vi "generate wave packet V3.vi"(7 "number of grid points":i32=300, 9 "z window":dbl=3.0, 11 "wavepacket in":T1={"R"=0.5, "wave number"=22.0, "delta k"=7.0, "radii vector"=[], "radial section"=[], "wave vector"=22.0, "wavepacket is"=TRUE} {"delta k" format="%#_3f"; "wave number" format="%#_3f"; "R" format="%#_3f"}) -> (1 "pond array out":cdb[][](array[numeric]), 2 "wavepacket array out":cdb[][](array[numeric]), 3 "wavepacket out":T1={"R"=0.5, "wave number"=22.0, "delta k"=7.0, "radii vector"=[], "radial section"=[], "wave vector"=22.0, "wavepacket is"=TRUE} {"delta k" format="%#_3f"; "wave number" format="%#_3f"; "R" format="%#_3f"})   [LabVIEW 2010]
uses:
  complex region.ctl
  wavepacket.ctl
panel:
  in  "complex region":T2={"max re"=5.161869466666667e-06, "min re"=5.176843333333334e-06, "max im"=-2.467216e-05, "min im"=-0.001573233, "delta re"=0.003211203, "delta im"=0.00165815, "center re"=0.0015485608400000002, "delta  z"=0.0015530530000000002+0.0i, "center im"=0.0, "center z"=0.0+0.0i, "d im"=0.0, "d re"=0.0, "d z"=0.0+0.0i}
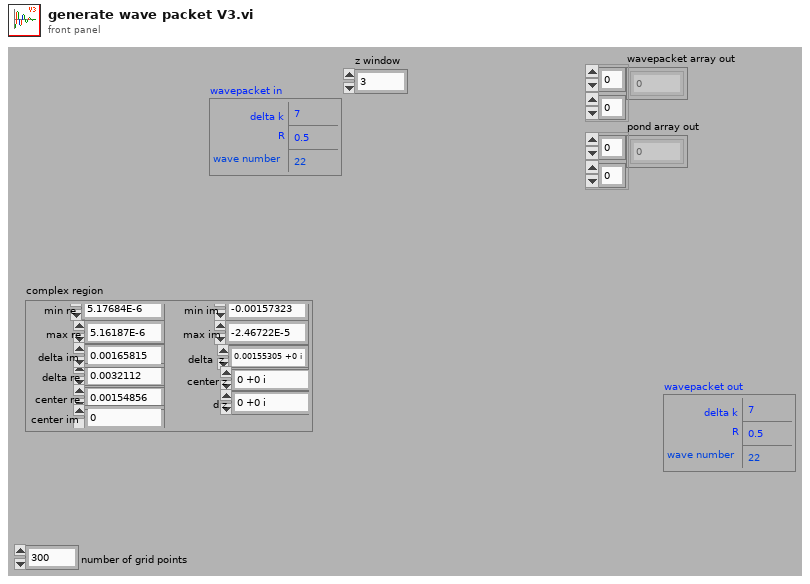
[diagram p1: front panel]
types:
  T1 = typedef "wavepacket.ctl" = cluster{"R":dbl, "wave number":dbl, "delta k":dbl, "radii vector":dbl[], "radial section":cdb[], "wave vector":dbl, "wavepacket is":bool}
  T2 = typedef "complex region.ctl" = cluster{"max re":dbl, "min re":dbl, "max im":dbl, "min im":dbl, "delta re":dbl, "delta im":dbl, "center re":dbl, "delta  z":cdb, "center im":dbl, "center z":cdb, "d im":dbl, "d re":dbl, "d z":cdb}
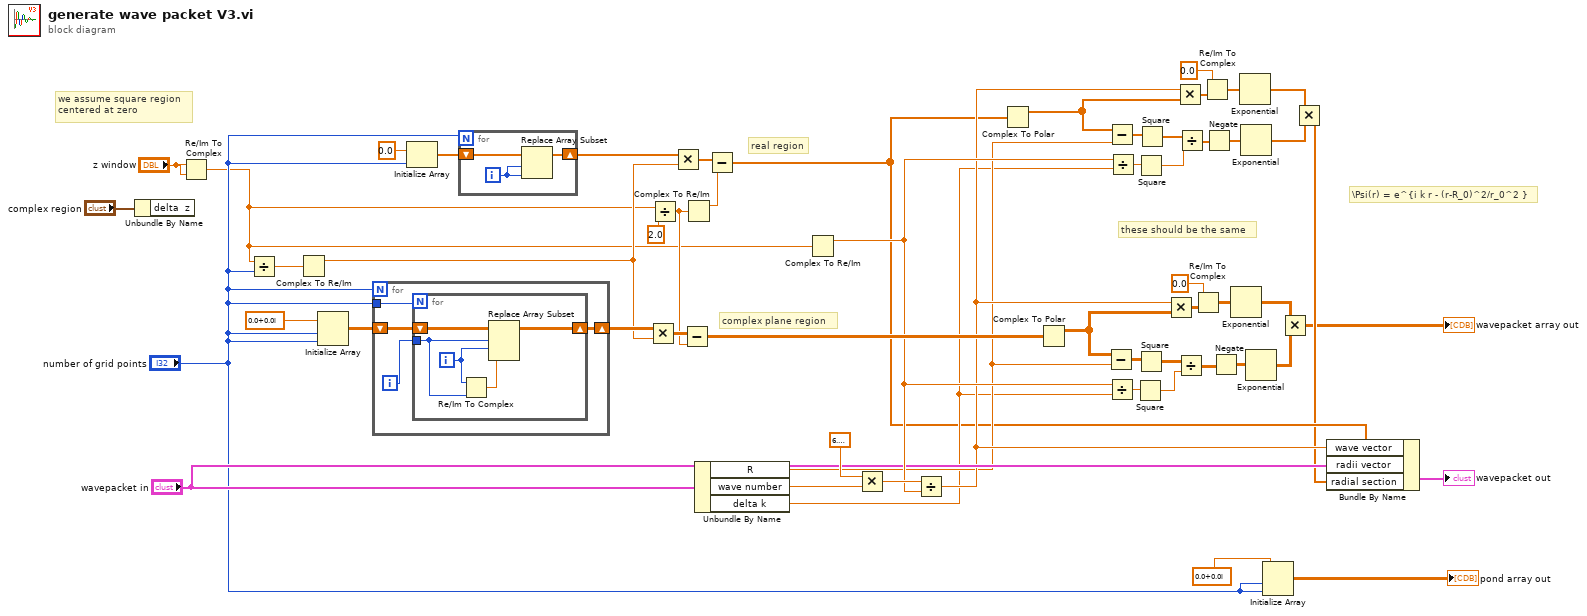
[diagram p0: block diagram]
diagram:
  # "complex plane region"
  # "real region"
  # "we assume square region\ncentered at zero"
  # "\\Psi(r) = e^{i k r - (r-R_0)^2/r_0^2 }"
  # "these should be the same"
  n1 = Unbundle By Name("complex region") -> ()  [unwired: 1 out]
  n2 = Re/Im To Complex(1:"z window", 2:"z window") -> (0:w1:cdb)
  n3 = Divide(x=w1, y="number of grid points") -> (x/y=w25:cdb)
  n4 = Complex To Re/Im(x + iy=w25) -> (x=w22:dbl)  [unwired: 1 out]
  n5 = Initialize Array(cdb 0.0+0.0i ("element"), "number of grid points", "number of grid points") -> (w28:cdb[][])
  n6 = for {
    N: "number of grid points" -> [_]
    tunnel: "number of grid points" -> [w59]
    shift-right: [w58] -> w23
    shift-left: w28 -> [w60]
    i -> [w57]
    n7 = for {
      N: w59 -> [_]
      shift-right: [w64] -> w58
      shift-left: w60 -> [w65]
      tunnel: w57 -> [w61]
      i -> [w62]
      n8 = Re/Im To Complex(1:w61, 2:w62) -> (0:w63:cdb)
      n9 = Replace Array Subset(array=w65, new element=w63, index (row)=w61, index (col)=w62) -> (w64:cdb[][])
    }
  }
  n10 = Initialize Array(0.0 ("element"), "number of grid points") -> (w33:dbl[])
  n11 = for {
    N: "number of grid points" -> [_]
    shift-right: [w67] -> w31
    shift-left: w33 -> [w68]
    i -> [w66]
    n12 = Replace Array Subset(array=w68, new element=w66, index=w66) -> (w67:dbl[])
  }
  n13 = Multiply(x=w23, y=w22) -> (x*y=w27:cdb[][])
  n14 = Divide(x=w1, y=2.0) -> (x/y=w24:cdb)
  n15 = Multiply(x=w31, y=w22) -> (x*y=w30:dbl[])
  n16 = Subtract(x=w27, y=w24) -> (x-y=w21:cdb[][])
  n17 = Complex To Re/Im(x + iy=w24) -> (x=w26:dbl)  [unwired: 1 out]
  n18 = Unbundle By Name("wavepacket in") -> ("R"=w11:dbl, "wave number"=w13:dbl, "delta k"=w10:dbl)
  n19 = Subtract(x=w30, y=w26) -> (x-y=w9:dbl[])
  n20 = Complex To Re/Im(x + iy=w1) -> (x=w15:dbl)  [unwired: 1 out]
  n21 = Multiply(x=6.283185307179586, y=w13) -> (x*y=w46:dbl)
  n22 = Divide(x=w46, y=w15) -> (x/y=w12:dbl)
  n23 = Complex To Polar(r * e^(i*theta)=w9) -> (r=w37:dbl[])  [unwired: 1 out]
  n24 = Complex To Polar(r * e^(i*theta)=w21) -> (r=w16:dbl[][])  [unwired: 1 out]
  n25 = Subtract(x=w16, y=w11) -> (x-y=w54:dbl[][])
  n26 = Subtract(x=w37, y=w11) -> (x-y=w44:dbl[])
  n27 = Divide(x=w15, y=w10) -> (x/y=w53:dbl)
  n28 = Divide(x=w15, y=w10) -> (x/y=w43:dbl)
  n29 = Square(x=w53) -> (x^2=w35:dbl)
  n30 = Square(x=w43) -> (x^2=w36:dbl)
  n31 = Square(x=w54) -> (x^2=w55:dbl[][])
  n32 = Square(x=w44) -> (x^2=w45:dbl[])
  n33 = Multiply(x=w12, y=w16) -> (x*y=w52:dbl[][])
  n34 = Multiply(x=w12, y=w37) -> (x*y=w42:dbl[])
  n35 = Divide(x=w55, y=w35) -> (x/y=w18:dbl[][])
  n36 = Divide(x=w45, y=w36) -> (x/y=w20:dbl[])
  n37 = Re/Im To Complex(1:w52, 2:0.0 ("x")) -> (0:w50:cdb[][])
  n38 = Re/Im To Complex(1:w42, 2:0.0 ("x")) -> (0:w40:cdb[])
  n39 = Negate(x=w20) -> (-x=w19:dbl[])
  n40 = Negate(x=w18) -> (-x=w17:dbl[][])
  n41 = Exponential(1:w50) -> (0:w48:cdb[][])
  n42 = Exponential(1:w40) -> (0:w38:cdb[])
  n43 = Exponential(1:w19) -> (0:w39:dbl[])
  n44 = Exponential(1:w17) -> (0:w49:dbl[][])
  n45 = Initialize Array(cdb 0.0+0.0i ("element"), "number of grid points", "number of grid points") -> (→"pond array out":cdb[][])
  n46 = Multiply(x=w49, y=w48) -> (x*y=→"wavepacket array out":cdb[][])
  n47 = Multiply(x=w39, y=w38) -> (x*y=w8:cdb[])
  n48 = Bundle By Name(cluster="wavepacket in", "wave vector"=w12, "radii vector"=w9, "radial section"=w8) -> (→"wavepacket out":T1)
